vi "Check ivision File Exist.vi"(8 "error in (no error)":errorcluster, 11 "SequenceEditorRoothPath":path) -> (0 "error out":errorcluster, 3 "file or folder exists?":bool)   [LabVIEW 2015]
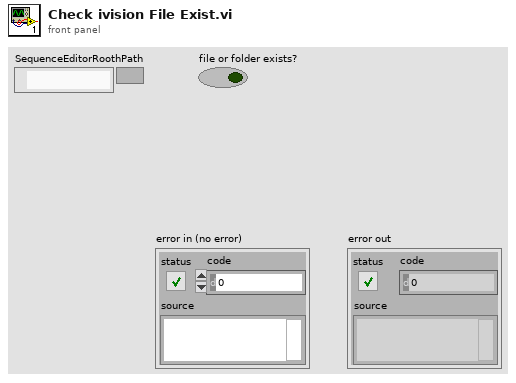
[diagram p1: front panel]
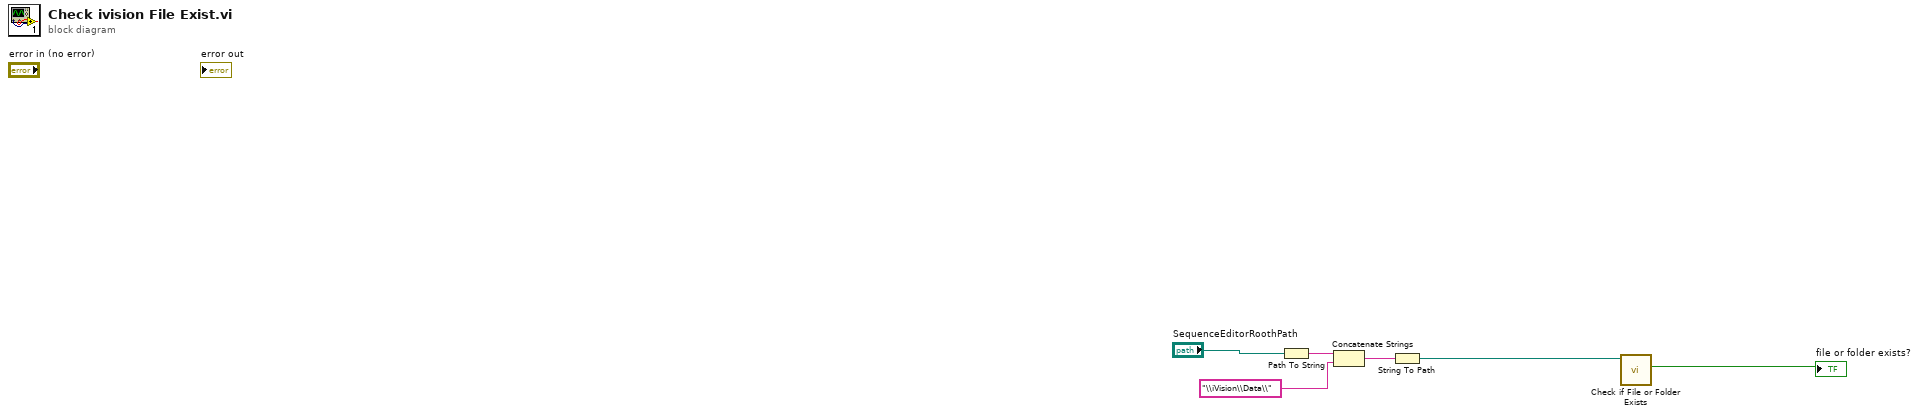
[diagram p0: block diagram]
diagram:
  n1 = Path To String(path="SequenceEditorRoothPath") -> (string=w4:string)
  n2 = Concatenate Strings(w4, "\\iVision\\Data\\") -> (w2:string)
  n3 = String To Path(string=w2) -> (path=w1:path)
  n4 = call <vilib>:"Check if File or Folder Exists.vi"("path"=w1) -> ("file or folder exists?"=→"file or folder exists?":bool)  [unwired: 8 in, 2 out]
